vi "projekt_LV.vi"() -> ()   [LabVIEW 2018]
uses:
  <vilib>/Instr/_visa.llb/VISA Configure Serial Port (Instr).vi
panel:
  in  "file path (use dialog)":path
  in  "stop":bool
  in  "VISA resource name":refnum<visa-resource-name>
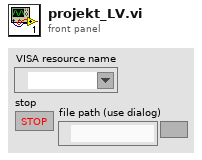
[diagram p1: front panel]
types:
  T1 = enum16{"open", "replace", "create", "open or create", "replace or create", "replace or create with confirmation"}
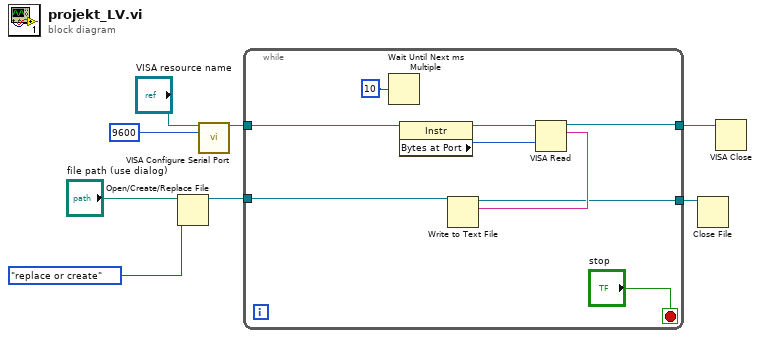
[diagram p0: block diagram]
diagram:
  n1 = Open/Create/Replace File(file path (use dialog)="file path (use dialog)", operation (0:open)=T1."replace or create") -> (refnum out=w2:refnum<file>)  [unwired: 4 in, 2 out]
  n2 = call-poly "VISA Configure Serial Port"("VISA resource name"="VISA resource name", "baud rate (9600)"=u32 9600) -> ("VISA resource name out"=w6:refnum<visa-resource-name>)  [unwired: 12 in, 1 out]
  n3 = while {
    tunnel: w6 -> [w12]
    tunnel: [w14] -> w5
    tunnel: w2 -> [w10]
    tunnel: [w9] -> w1
    stop <- "stop" stop-if-true
    n4 = Wait Until Next ms Multiple(millisecond multiple=u32 10) -> ()  [unwired: 1 out]
    n5 = property class="Instr"(reference=w12) -> (reference out=w16:refnum<visa-resource-name>, "Bytes at Port"=w13:u32)  [unwired: 1 in, 1 out]
    n6 = VISA Read(VISA resource name=w16, byte count=w13) -> (VISA resource name out=w14:refnum<visa-resource-name>, read buffer=w11:string)  [unwired: 1 in, 2 out]
    n7 = Write to Text File(file (use dialog)=w10, text=w11) -> (refnum out=w9:refnum<file>)  [unwired: 2 in, 2 out]
  }
  n8 = Close File(refnum=w1) -> ()  [unwired: 1 in, 2 out]
  n9 = VISA Close(VISA resource name=w5) -> ()  [unwired: 1 in, 1 out]
